vi "Step Result Status Convert.vi"(1 "Result":T1) -> (0 "Result String":string)   [LabVIEW 2015, in "JsonReportPlugin.lvclass"]
uses:
  JsonReportPlugin.lvclass
  Core/Step/STEP_STATUS.ctl
  Core/Step.lvclass
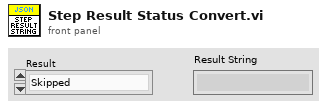
[diagram p1: front panel]
types:
  T1 = typedef "Step.lvclass/STEP_STATUS.ctl" = enum16{"Skipped", "Done", "Passed", "Failed", "Error"}
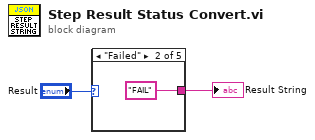
[diagram p0: block diagram]
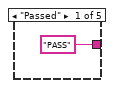
[diagram p2: hidden frame]
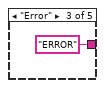
[diagram p3: hidden frame]
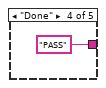
[diagram p4: hidden frame]
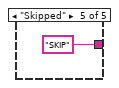
[diagram p5: hidden frame]
diagram:
  n1 = case shown="\"Failed\"" "Result" {
    tunnel: ["PASS" "FAIL" "ERROR" "PASS" "SKIP"] -> w1
    frame "Passed" {
    }
    frame "Failed" {
    }
    frame "Error" {
    }
    frame "Done" {
    }
    frame "Skipped" {
    }
  }
  "Result String" <- w1
